vi "D Printer Setup.vi"(5 "Address(5)":u32=5, 6 "Baud Rate(9600)":u32(ring)=3 items=["1200", "2400", "4800", "9600", "19200"], 7 "Port(Parallel:0)":u16(ring) items=["Parallel", "Serial", "GPIB"], 8 "error in (no error)":errorcluster, 9 "Type(Plotter)":u16(ring) items=["DeskJet", "Epson ESC/P2", "LaserJet", "PaintJet", "ThinkJet"], 10 "Handshake Mode(F:Xon-Xoff)":bool, 11 "VISA resource name":refnum<visa-resource-name>) -> (0 "error out":errorcluster, 3 "VISA resource name out":refnum<visa-resource-name>)   [LabVIEW 2018, in "Agilent 87XX Series.lvlib"]
doc: "Sets up configuration information for the printer. Only works on the HP8753D."
uses:
  Agilent 87XX Series.lvlib
panel:
  # "DTR-DSR"
  # "Xon-Xoff"
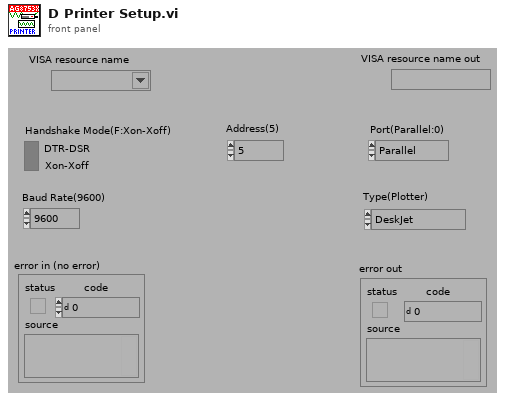
[diagram p1: front panel]
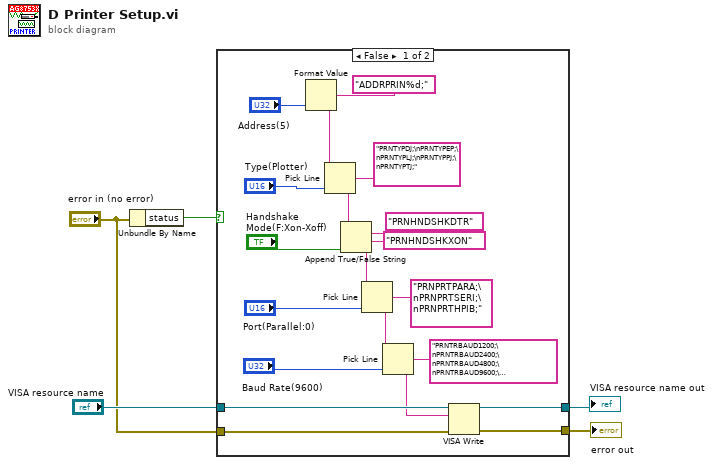
[diagram p0: block diagram]
diagram:
  n1 = Unbundle By Name("error in (no error)") -> ("status"=w5:bool)
  n2 = case shown="False" w5 {
    tunnel: [w25 w26] -> w4
    tunnel: "VISA resource name" -> [w24 w27]
    tunnel: "error in (no error)" -> [w23 w26]
    tunnel: [w22 w27] -> w1
    frame False {
      n3 = Format Value(format string="ADDRPRIN%d;", value (0)="Address(5)") -> (output string=w6:string)  [unwired: 1 in]
      n4 = Pick Line(string ("")=w6, multi-line string="PRNTYPDJ;\nPRNTYPEP;\nPRNTYPLJ;\nPRNTYPPJ;\nPRNTYPTJ;", line index="Type(Plotter)") -> (output string=w13:string)
      n5 = Append True/False String(1:"Handshake Mode(F:Xon-Xoff)", 2:"PRNHNDSHKXON", 3:"PRNHNDSHKDTR", 4:w13) -> (0:w12:string)
      n6 = Pick Line(string ("")=w12, multi-line string="PRNPRTPARA;\nPRNPRTSERI;\nPRNPRTHPIB;", line index="Port(Parallel:0)") -> (output string=w19:string)
      n7 = Pick Line(string ("")=w19, multi-line string="PRNTRBAUD1200;\nPRNTRBAUD2400;\nPRNTRBAUD4800;\nPRNTRBAUD9600;\nPRNTRBAUD19200;", line index="Baud Rate(9600)") -> (output string=w9:string)
      n8 = VISA Write(VISA resource name=w24, write buffer=w9, error in (no error)=w23) -> (VISA resource name out=w22:refnum<visa-resource-name>, error out=w25:errorcluster)  [unwired: 1 out]
    }
    frame True {
    }
  }
  "VISA resource name out" <- w1
  "error out" <- w4
